vi "8.反馈节点.vi"() -> ()   [LabVIEW 2019]
uses:
  <vilib>/Platform/TimedLoop/XDataNode/timing_clust.ctl
  <vilib>/Platform/TimedLoop/XDataNode/nitl_modes.ctl
  <vilib>/Platform/TimedLoop/XDataNode/wakeup.ctl
  <vilib>/rvi/Emulation/niFpgaSctlEmulationGetInTimedLoop.vi
  <vilib>/rvi/Emulation/niFpgaEmulationReportErrorSimple.vi
  <vilib>/rvi/Emulation/niFpgaGetClockAttributes.vi
  <vilib>/rvi/Emulation/niFpgaCriticalErrorInLSC.vi
  <vilib>/rvi/eio/common/nirviEmuTemplateMethod_errors.vi
  <vilib>/Platform/TimedLoop/XDataNode/XDataNode.xnode
  <vilib>/eio/EIONode/EIONode.xnode
  <vilib>/Platform/TimedLoop/XDataNode/XDNodeRunTimeDep.lvlib
panel:
  out "Counters":u8
  out "当前嘀嗒数":u64
  in  "去抖动":u64=40000
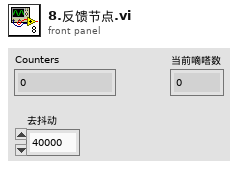
[diagram p1: front panel]
types:
  T1 = typedef "XDNodeRunTimeDep.lvlib/timing_clust.ctl" = cluster{"Expected End [f-1]":u64, "Actual End [f-1]":u64, "Finished Late? [f-1]":bool, "Expected End [i-1]":u64, "Actual End [i-1]":u64, "Finished Late? [i-1]":bool, "Expected Start [i]":u64, "Actual Start [i]":u64, "Expected Start [f]":u64, "Actual Start [f]":u64, "Source Name":string, "Structure Name":string, "Period":i64, "Deadline":i64, "Offset":i64, "Start":i64, "Priority":i32, "Timeout":i32, "Mode":T2, "Wakeup Reason":T3, "Error":errorcluster, "Source Type":string, "Secondary Source Type":string, "Global End Time":u64, "Global Start Time":u64, "Frame Duration":u64, "Iteration Duration":u64, "Assigned CPU":i32, "I/O Scan Engine Mode":u32}
  T2 = typedef "XDNodeRunTimeDep.lvlib/nitl_modes.ctl" = enum32{"No Change", "Process missed periods, maintain original phase", "Discard missed periods, maintain original phase", "Process missed periods, ignore original phase", "Discard missed periods, ignore original phase"}
  T3 = typedef "XDNodeRunTimeDep.lvlib/wakeup.ctl" = enum32{"Normal", "Aborted", "Asynchronous wakeup", "Timing source error", "Timed loop error", "Timeout"}
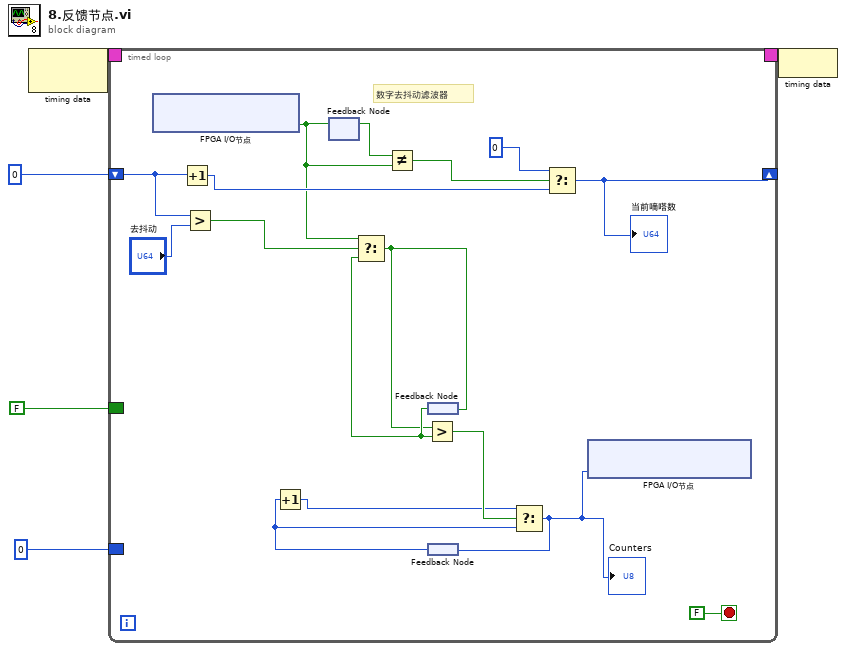
[diagram p0: block diagram]
diagram:
  n1 = node-c288() -> (w5:T1)  [unwired: 1 in]
  n2 = timed-loop {
    timing: w5 -> [_]
    timing-out: [_] -> w4
    shift-right: [w13] -> _
    shift-left: u64 0 -> [w12]
    border: u8 0 -> [_]
    border: FALSE -> [_]
    stop <- FALSE stop-if-true
    # "数字去抖动滤波器"
    n3 = xnode "FPGA I/O节点"() -> ("ConnectorA/DIO1"=w7:bool)  [unwired: 1 in, 1 out]
    n4 = Increment(x=w12) -> (x+1=w14:u64)
    n5 = Greater?(x=w12, y="去抖动") -> (0:w10:bool)
    n6 = feedback-in #1(w7) -> ()
    n7 = feedback #1() -> (w6:bool)  [unwired: 1 in]
    n8 = Not Equal?(x=w6, y=w7) -> (x != y?=w16:bool)
    n9 = feedback #2() -> (w9:bool)
    n10 = Select(t=w7, s=w10, f=w9) -> (s? t:f=w8:bool)
    n11 = Greater?(x=w8, y=w9) -> (0:w20:bool)
    n12 = feedback-in #2(w8) -> ()
    n13 = feedback #3() -> (w18:u8)
    n14 = Increment(x=w18) -> (x+1=w19:u8)
    n15 = Select(t=w19, s=w20, f=w18) -> (s? t:f=w17:u8)
    "Counters" <- w17
    n16 = feedback-in #3(w17) -> ()
    n17 = Select(t=u64 0, s=w16, f=w14) -> (s? t:f=w13:u64)
    "当前嘀嗒数" <- w13
    n18 = xnode "FPGA I/O节点"("ConnectorA/DIO15:8"=w17) -> ()  [unwired: 1 in, 1 out]
  }
  n19 = node-c288(w4) -> ()
